vi "Configure Sliding Window Trigger 20221110.vi"(0 "device session in":refnum<class "Device Session.lvclass">, 5 "Sliding Window Triggers (FXP)":T1[](array[typedef]), 7 "ResetTrig":bool, 11 "error in":errorcluster) -> (4 "device session out":refnum<class "Device Session.lvclass">, 15 "error out":errorcluster)   [LabVIEW 2021, in "Device Session.lvclass"]
doc: "Configures the edge trigger for the selected channel. You can specify the trigger level, hysteresis, and trigger slope.\n\n<B>Input Parameters</B>\n\n<B>device session in</B> is a reference to the Device Session object, which contains a session to each instrument design library used in this sample project. This parameter is obtained from the 'Open Session' VI.\n\n<B>trigger source</B> specifies the channel to monitor for trigger conditions.\n\n<B>trigger slope</B> specifies whether the oscilloscope should trigger on a rising edge or a falling edge.\n\n<B>trigger level (V)</B> specifies the voltage threshold for the trigger.\n\n<B>hysteresis (%fs)</B> specifies in volts the size of the hysteresis window on either side of the specified 'level'. The oscilloscope triggers when the 'trigger source' signal passes through the 'hysteresis level' you specify with this parameter, has the specified 'trigger slope', and passes through the specified 'level'.\n\n<B>instance</B> specifies either instance A or B of the trigger to use.\n\n<B>error in</B> describes error conditions that occur before this node runs. This input provides standard 'error in' functionality.\n\n<B>Output Parameters</B>\n\n<B>device session out</B> passes a reference to the session to the next VI.\n\n<B>error out</B> contains error information. This output provides standard 'error out' functionality."
uses:
  Device Session.lvclass
  Clusts/ChannelWindowClust.ctl
  Device Session.lvclass/Device Session.ctl
  Clusts/AllWindowsClust.ctl
  <vilib>/Utility/error.llb/Error Cluster From Error Code.vi
  <vilib>/rvi/errors/niLvFpgaAdjustHostInterfaceError.vi
  <vilib>/rvi/interface/nirviReadWriteControl/nirviReadWriteControl.xnode
  FPGA Refnum.ctl
  NiFpgaLv.dll
  <vilib>/rvi/interface/Simulation/niFpgaSimulationCallBeginRW.vi
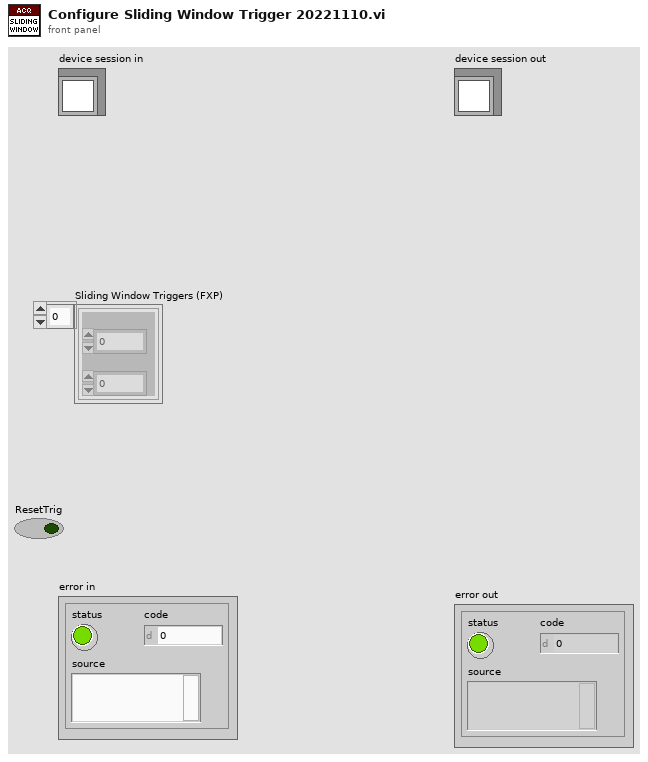
[diagram p1: front panel]
types:
  T1 = typedef "ChannelWindowClust.ctl" = cluster{"HalfRange":fxp<+/-,18,5>, "StartCenter":fxp<+/-,18,5>}
  T2 = typedef "AllWindowsClust.ctl" = cluster{"0":T1, "1":T1, "2":T1, "3":T1, "4":T1, "5":T1, "6":T1, "7":T1}
  T3 = typedef "Device Session.lvclass/Device Session Object.ctl" = cluster{"fpga reference":T4, "reg bus":refnum<class "niInstr FIFO Register Bus v1 Host.lvclass">, "subsystem map":refnum<class "niInstr Subsystem Map v1 Host.lvclass">, "cal data":refnum<class "niHSAI Cal Data v1 Host.lvclass">, "config":refnum<class "niHSAI Group A Config v1 Host.lvclass">, "acquisition":refnum<class "niInstr Multirecord Acquisition v1 Host.lvclass">, "number of selected acq channels":u8, "selected acq channels":bool[], "number of channels":u32, "configured channels":bool[], "acq configuration":cluster{"number of samples":u64, "number of records":u64, "pretrigger samples":u64}, "actual channel configuration":T5[], "sample clock rate (Hz)":dbl, "scaling coefficients":T9[]}
  T4 = typedef "Device Session.lvclass/FPGA Refnum.ctl" = refnum<k20>
  T5 = typedef "niHSAI Types v1 Host.lvlib/Channel Configuration.ctl" = cluster{"channel":u32, "coupling":T6, "impedance":T7, "bandwidth":T8, "vertical range":dbl, "vertical offset":dbl}
  T6 = typedef "niHSAI Types v1 Host.lvlib/Coupling.ctl" = enum8{"Default", "DC", "AC"}
  T7 = typedef "niHSAI Types v1 Host.lvlib/Impedance.ctl" = enum8{"Default", "1 mega ohm", "50 ohm"}
  T8 = typedef "niHSAI Types v1 Host.lvlib/Bandwidth.ctl" = enum8{"Default", "Full Bandwidth", "Anti-alias Filter", "150 MHz"}
  T9 = typedef "niInstr Multirecord Acquisition v1 Host.lvclass/Scaling Coefficient.ctl" = cluster{"gain":dbl, "offset":dbl}
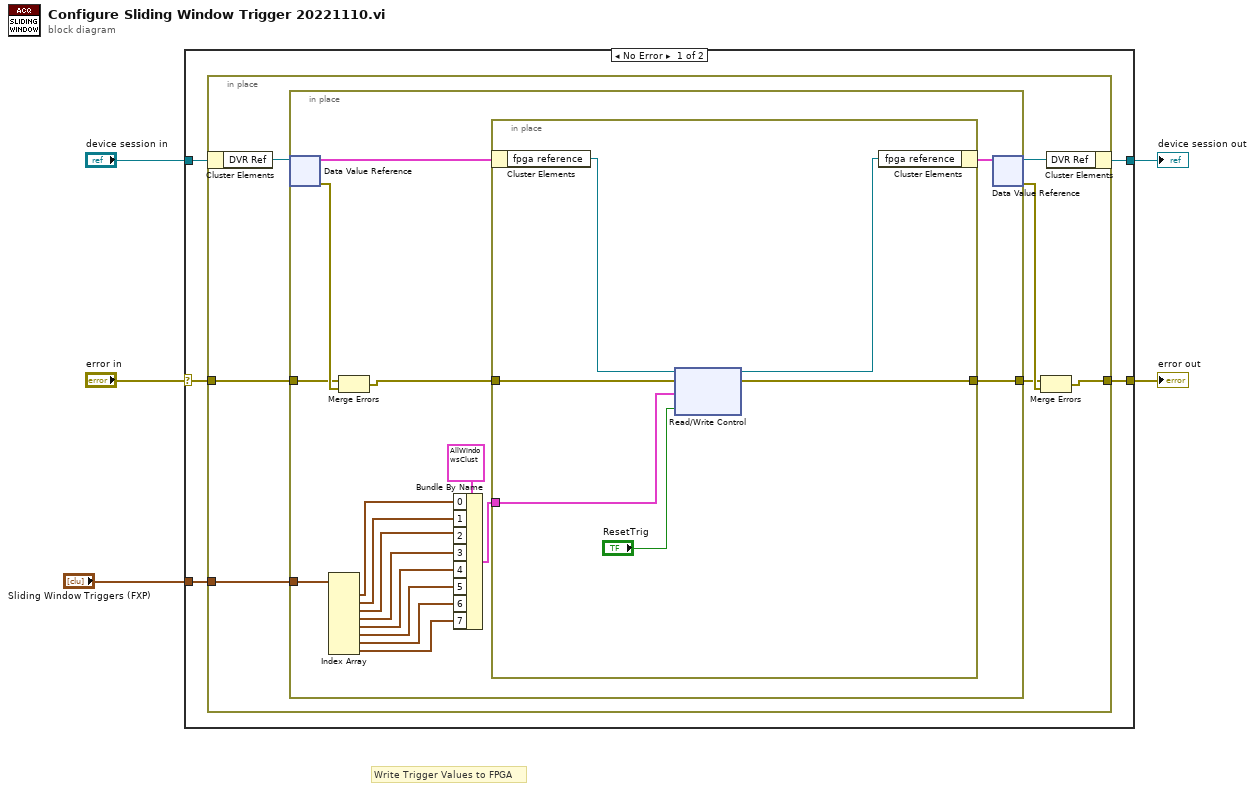
[diagram p0: block diagram]
diagram:
  # "Write Trigger Values to FPGA"
  n1 = case shown="No Error" "error in" {
    selector: "error in" -> [w10 w42]
    tunnel: "device session in" -> [w8 w41]
    tunnel: [w7 w41] -> w4
    tunnel: [w9 w42] -> w5
    tunnel: "Sliding Window Triggers (FXP)" -> [w6 _]
    frame No Error {
      n2 = in-place {
        in-place-border: w10 -> [w17]
        in-place-border: [w14] -> w9
        in-place-border: w6 -> [w11]
        n3 = in-place-cluster #1(w8) -> ("DVR Ref"=w13:refnum<data-value>)
        n4 = in-place {
          in-place-border: w17 -> [w33]
          in-place-border: [w32] -> w15
          in-place-border: w11 -> [w26]
          n5 = in-place-dvr #2(w13) -> (w30:T3, w34:errorcluster)
          n6 = Index Array(array=w26) -> (element #1=w25:T1, element #2=w24:T1, element #3=w23:T1, element #4=w22:T1, element #5=w21:T1, element #6=w20:T1, element #7=w19:T1, element #8=w18:T1)  [unwired: 8 in]
          n7 = Merge Errors(w33, w34) -> (w31:errorcluster)
          n8 = Bundle By Name(cluster=T2 {"0"={"HalfRange"=0.0, "StartCenter"=0.0}, "1"={"HalfRange"=0.0, "StartCenter"=0.0}, "2"={"HalfRange"=0.0, "StartCenter"=0.0}, "3"={"HalfRange"=0.0, "StartCenter"=0.0}, "4"={"HalfRange"=0.0, "StartCenter"=0.0}, "5"={"HalfRange"=0.0, "StartCenter"=0.0}, "6"={"HalfRange"=0.0, "StartCenter"=0.0}, "7"={"HalfRange"=0.0, "StartCenter"=0.0}} ("AllWindows"), "0"=w25, "1"=w24, "2"=w23, "3"=w22, "4"=w21, "5"=w20, "6"=w19, "7"=w18) -> (w27:T2)
          n9 = in-place {
            in-place-border: [w40] -> w32
            in-place-border: w31 -> [w39]
            in-place-border: w27 -> [w35]
            n10 = in-place-cluster #3(w30) -> ("fpga reference"=w38:T4)
            n11 = xnode "Read/Write Control"("FPGA VI Reference In"=w38, "error in"=w39, "UserTrig"=w35, "ResetTrig"="ResetTrig") -> ("FPGA VI Reference Out"=w37:T4, "error out"=w40:errorcluster)
            n12 = in-place-cluster #3("fpga reference"=w37) -> (w29:T3)
          }
          n13 = in-place-dvr #2(w29) -> (w12:refnum<data-value>, w16:errorcluster)
        }
        n14 = Merge Errors(w15, w16) -> (w14:errorcluster)
        n15 = in-place-cluster #1("DVR Ref"=w12) -> (w7:refnum<class "Device Session.lvclass">)
      }
    }
    frame Error {
    }
  }
  "error out" <- w5
  "device session out" <- w4
